vi "Array Of Variants To Variant.vi"(4 "Type Enum [auto]":T1, 6 "Variant":variant, 8 "error in (no error)":errorcluster, 9 "Elements":variant[](array[variant]), 11 "Registry Variant Accessor in":refnum<class "CConfig Variant Accessor.lvclass">) -> (0 "error out":errorcluster, 2 "Variant":variant, 3 "Registry Variant Accessor out":refnum<class "CConfig Variant Accessor.lvclass">)   [LabVIEW 2013, in "CConfig Variant Accessor.lvclass"]
doc: "Copyright 2018, Carya Automatisering, Wiebe Walstra."
uses:
  CConfig Variant Accessor.lvclass
  <vilib>/Utility/VariantDataType/Type.ctl
  <vilib>/Utility/VariantDataType/VariantType.lvlib
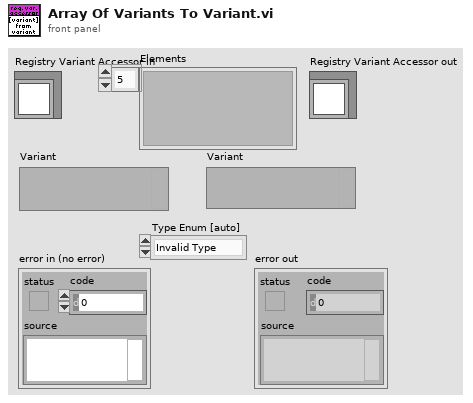
[diagram p1: front panel]
types:
  T1 = typedef "VariantType.lvlib/Type.ctl" = enum8{"Invalid Type", "Void", "I8", "I16", "I32", "I64", "U8", "U16", "U32", "U64", "Single Float", "Double Float", "Extended Float", "Single Complex", "Double Complex", "Extended Complex", "Enum U8", "Enum U16", "Enum U32", "Enum U64", "Single Float With Unit", "Double Float With Unit", "Extended Float With Unit", "Single Complex with Unit", "Double Complex with Unit", "Extended Complex with Unit", "Boolean", "String", "Path", "Picture", "Tag", "Array", "Cluster", "Variant", "LV Variant", "Waveform", "Timestamp", "Digital Waveform", "Digital Data", "ExpressData", "Refnum", "External Data", "VI", "Poly VI", "LabVIEW Class Instance", "Fixed Point"}
  T2 = cluster{"Major":u16, "Minor":u16, "Fix":u16, "Build":u16}[]
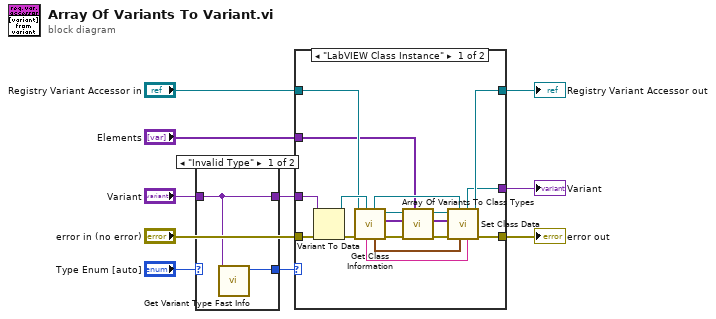
[diagram p0: block diagram]
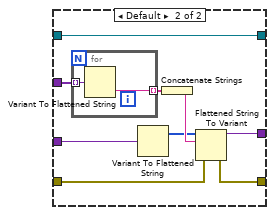
[diagram p2: hidden frame]
diagram:
  n1 = case shown="\"Invalid Type\"" "Type Enum [auto]" {
    selector: "Type Enum [auto]" -> [_ w14]
    tunnel: "Variant" -> [w11 w13]
    tunnel: [w12 w14] -> w3
    tunnel: [w11 w13] -> w4
    frame "Invalid Type" {
      n2 = call "Get Variant Type Fast Info.vi"("Variant"=w11) -> ("Type Enum"=w12:T1)  [unwired: 6 in, 4 out]
    }
    frame Default {
    }
  }
  n3 = case shown="\"LabVIEW Class Instance\"" w3 {
    tunnel: [w28 w41] -> w10
    tunnel: "Elements" -> [w21 w37]
    tunnel: "error in (no error)" -> [w25 w36]
    tunnel: [w31 w35] -> w7
    tunnel: w4 -> [w23 w34]
    tunnel: "Registry Variant Accessor in" -> [w22 w33]
    tunnel: [w32 w33] -> w1
    frame "LabVIEW Class Instance" {
      n4 = Variant To Data(error in=w25, Variant=w23) -> (data=w26:refnum<class>, error out=w24:errorcluster)  [unwired: 1 in]
      n5 = call "Get Class Information.vi"("Object"=w26, "error in (no error)"=w24, "CConfig Variant Accessor in"=w22) -> ("error out"=w17:errorcluster, "Class default data"=w16:variant[], "CConfig Variant Accessor out"=w15:refnum<class "CConfig Variant Accessor.lvclass">, "Class versions"=w30:T2, "Object (dup)"=w27:refnum<class>, "Class name"=w29:string)  [unwired: 3 in]
      n6 = call-dynamic "Array Of Variants To Class Types.vi"("Elements"=w21, "error in (no error)"=w17, "Class types"=w16, "Registry Variant Accessor in"=w15) -> ("error out"=w18:errorcluster, "Class types"=w20:variant[], "Registry Variant Accessor out"=w19:refnum<class "CConfig Variant Accessor.lvclass">)  [unwired: 5 in]
      n7 = call "Set Class Data.vi"("Class name"=w29, "Class versions"=w30, "Object"=w27, "error in (no error)"=w18, "Class default data"=w20, "CConfig Variant Accessor in"=w19) -> ("error out"=w31:errorcluster, "CConfig Variant Accessor out"=w32:refnum<class "CConfig Variant Accessor.lvclass">, "Object (dup)"=w28:refnum<class>)  [unwired: 3 in]
    }
    frame Default {
      n8 = for {
        tunnel: [w43] -> w40 mode=indexing
        tunnel: w37 -> [w42] mode=indexing
        n9 = Variant To Flattened String(Variant=w42) -> (data string=w43:string)  [unwired: 1 out]
      }
      n10 = Variant To Flattened String(Variant=w34) -> (1:w38:i16[])  [unwired: 1 out]
      n11 = Concatenate Strings(w40) -> (w39:string)
      n12 = Flattened String To Variant(4:w36, 6:w39, 7:w38) -> (0:w35:errorcluster, 3:w41:variant)
    }
  }
  "error out" <- w7
  "Registry Variant Accessor out" <- w1
  "Variant" <- w10
